vi "Three part faster sub live note on off.vi"() -> ()   [LabVIEW 2009]
uses:
  <vilib>/vision/Image Controls.llb/IMAQ Image.ctl
  <vilib>/userDefined/High Color/IMAQdx.ctl
  <vilib>/Instr/_visa.llb/VISA Configure Serial Port (Instr).vi
  <vilib>/vision/NI_Vision_Development_Module.lvlib
  <vilib>/vision/driver/NI_Vision_Acquisition_Software.lvlib
panel:
  in  "Drum Notes":bool
  out "Image 2":T1(plugin-control)
  in  "VISA resource name":refnum<visa-resource-name>
  out "number":u8 format="%b"
  out "decimal integer string":string
  out "decimal integer string 2":string
  out "decimal integer string 3":string
  out "number 2":u8 format="%b"
  out "number 3":u8 format="%b"
  out "Drum Cluster":T2
  out "Guitar Cluster":T3
  out "Bass Cluster":T4
  in  "Camera":T5="cam0"
  in  "Orange Bass":T6={"Global Rectangle"=[220, 302, 227, 392], "Contours"=[{"ID"=enum."External", "Type"=2, "Coordinates"=[226, 391, 220, 302]}]} {"Contours"."Type" items=["No Selection", "Point", "Line", "Rectangle", "Oval", "Polygon", "Freehand Region", "Annulus", "Unused2", "Unused3", "Broken Line", "Freehand Line", "Rotated Rectangle"]}
  in  "Blue Bass":T6={"Global Rectangle"=[192, 292, 199, 386], "Contours"=[{"ID"=enum."External", "Type"=2, "Coordinates"=[192, 385, 198, 292]}]} {"Contours"."Type" items=["No Selection", "Point", "Line", "Rectangle", "Oval", "Polygon", "Freehand Region", "Annulus", "Unused2", "Unused3", "Broken Line", "Freehand Line", "Rotated Rectangle"]}
  in  "playtime":dbl=90.0
  in  "Orange Guitar":T6={"Global Rectangle"=[587, 282, 628, 378], "Contours"=[{"ID"=enum."External", "Type"=2, "Coordinates"=[627, 377, 587, 282]}]} {"Contours"."Type" items=["No Selection", "Point", "Line", "Rectangle", "Oval", "Polygon", "Freehand Region", "Annulus", "Unused2", "Unused3", "Broken Line", "Freehand Line", "Rotated Rectangle"]}
  in  "Yellow Guitar":T6={"Global Rectangle"=[546, 282, 563, 376], "Contours"=[{"ID"=enum."External", "Type"=2, "Coordinates"=[562, 375, 546, 282]}]} {"Contours"."Type" items=["No Selection", "Point", "Line", "Rectangle", "Oval", "Polygon", "Freehand Region", "Annulus", "Unused2", "Unused3", "Broken Line", "Freehand Line", "Rotated Rectangle"]}
  in  "Green Guitar":T6={"Global Rectangle"=[498, 284, 505, 376], "Contours"=[{"ID"=enum."External", "Type"=2, "Coordinates"=[498, 375, 504, 284]}]} {"Contours"."Type" items=["No Selection", "Point", "Line", "Rectangle", "Oval", "Polygon", "Freehand Region", "Annulus", "Unused2", "Unused3", "Broken Line", "Freehand Line", "Rotated Rectangle"]}
  in  "Blue Guitar":T6={"Global Rectangle"=[569, 290, 594, 372], "Contours"=[{"ID"=enum."External", "Type"=2, "Coordinates"=[593, 371, 569, 290]}]} {"Contours"."Type" items=["No Selection", "Point", "Line", "Rectangle", "Oval", "Polygon", "Freehand Region", "Annulus", "Unused2", "Unused3", "Broken Line", "Freehand Line", "Rotated Rectangle"]}
  in  "Red Guitar":T6={"Global Rectangle"=[526, 284, 530, 370], "Contours"=[{"ID"=enum."External", "Type"=2, "Coordinates"=[529, 369, 526, 284]}]} {"Contours"."Type" items=["No Selection", "Point", "Line", "Rectangle", "Oval", "Polygon", "Freehand Region", "Annulus", "Unused2", "Unused3", "Broken Line", "Freehand Line", "Rotated Rectangle"]}
  in  "Green Bass":T6={"Global Rectangle"=[100, 292, 131, 371], "Contours"=[{"ID"=enum."External", "Type"=2, "Coordinates"=[100, 370, 130, 292]}]} {"Contours"."Type" items=["No Selection", "Point", "Line", "Rectangle", "Oval", "Polygon", "Freehand Region", "Annulus", "Unused2", "Unused3", "Broken Line", "Freehand Line", "Rotated Rectangle"]}
  in  "Red Bass":T6={"Global Rectangle"=[129, 294, 154, 376], "Contours"=[{"ID"=enum."External", "Type"=2, "Coordinates"=[129, 375, 153, 294]}]} {"Contours"."Type" items=["No Selection", "Point", "Line", "Rectangle", "Oval", "Polygon", "Freehand Region", "Annulus", "Unused2", "Unused3", "Broken Line", "Freehand Line", "Rotated Rectangle"]}
  in  "Yellow Bass":T6={"Global Rectangle"=[160, 295, 175, 378], "Contours"=[{"ID"=enum."External", "Type"=2, "Coordinates"=[160, 377, 174, 295]}]} {"Contours"."Type" items=["No Selection", "Point", "Line", "Rectangle", "Oval", "Polygon", "Freehand Region", "Annulus", "Unused2", "Unused3", "Broken Line", "Freehand Line", "Rotated Rectangle"]}
  out "Image Dst Out":T1
  in  "stop":bool
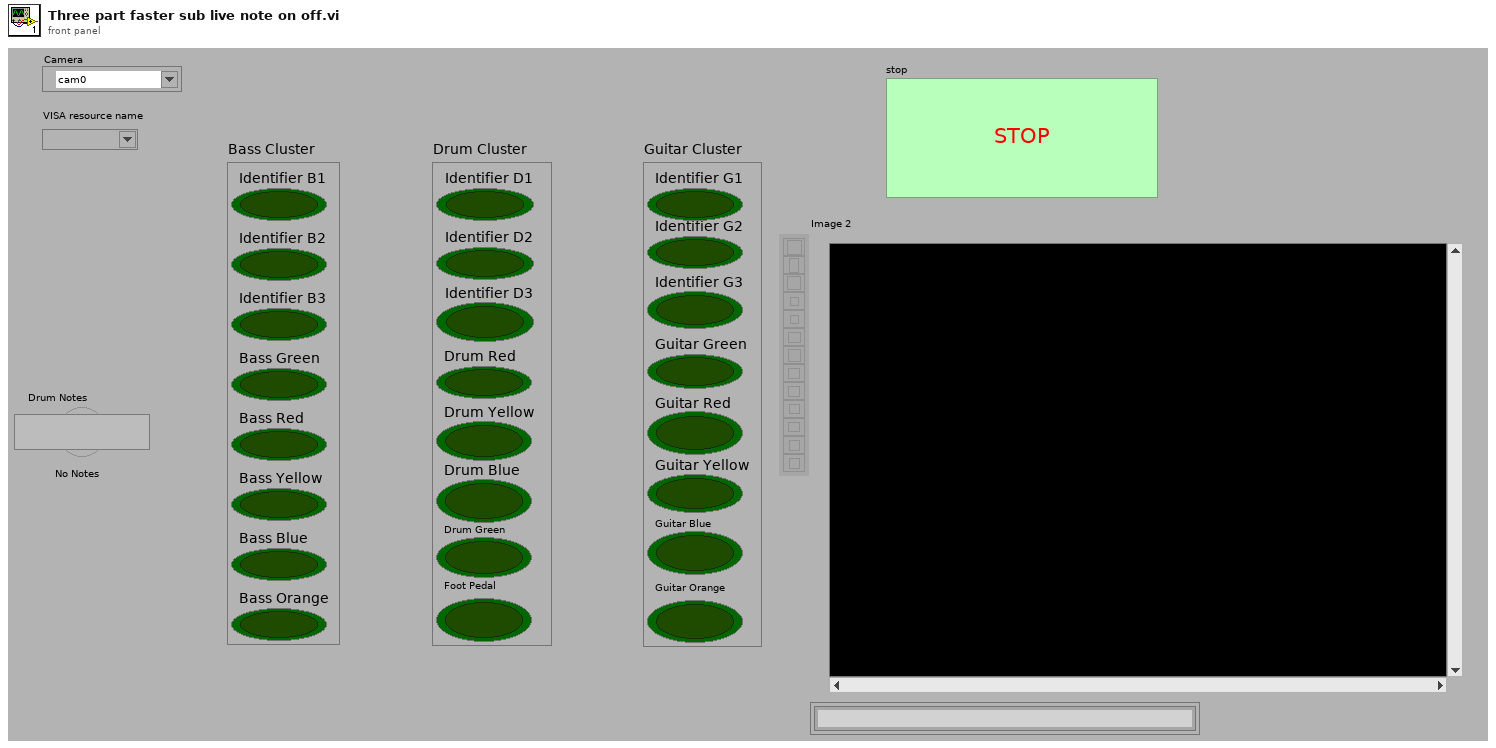
[diagram p1: front panel]
types:
  T1 = typedef "IMAQ Image.ctl" = refnum<image>
  T2 = cluster{"Identifier D1":bool, "Identifier D2":bool, "Identifier D3":bool, "Drum Red":bool, "Drum Yellow":bool, "Drum Blue":bool, "Drum Green":bool, "Foot Pedal":bool}
  T3 = cluster{"Identifier G1":bool, "Identifier G2":bool, "Identifier G3":bool, "Guitar Green":bool, "Guitar Red":bool, "Guitar Yellow":bool, "Guitar Blue":bool, "Guitar Orange":bool}
  T4 = cluster{"Identifier B1":bool, "Identifier B2":bool, "Identifier B3":bool, "Bass Green":bool, "Bass Red":bool, "Bass Yellow":bool, "Bass Blue ":bool, "Bass Orange":bool}
  T5 = typedef "IMAQdx.ctl" = refnum<k21>
  T6 = cluster{"Global Rectangle":i32[], "Contours":cluster{"ID":enum32{"External", "Internal"}, "Type":u32, "Coordinates":i32[]}[]}
  T7 = typedef "Image Type" = u32
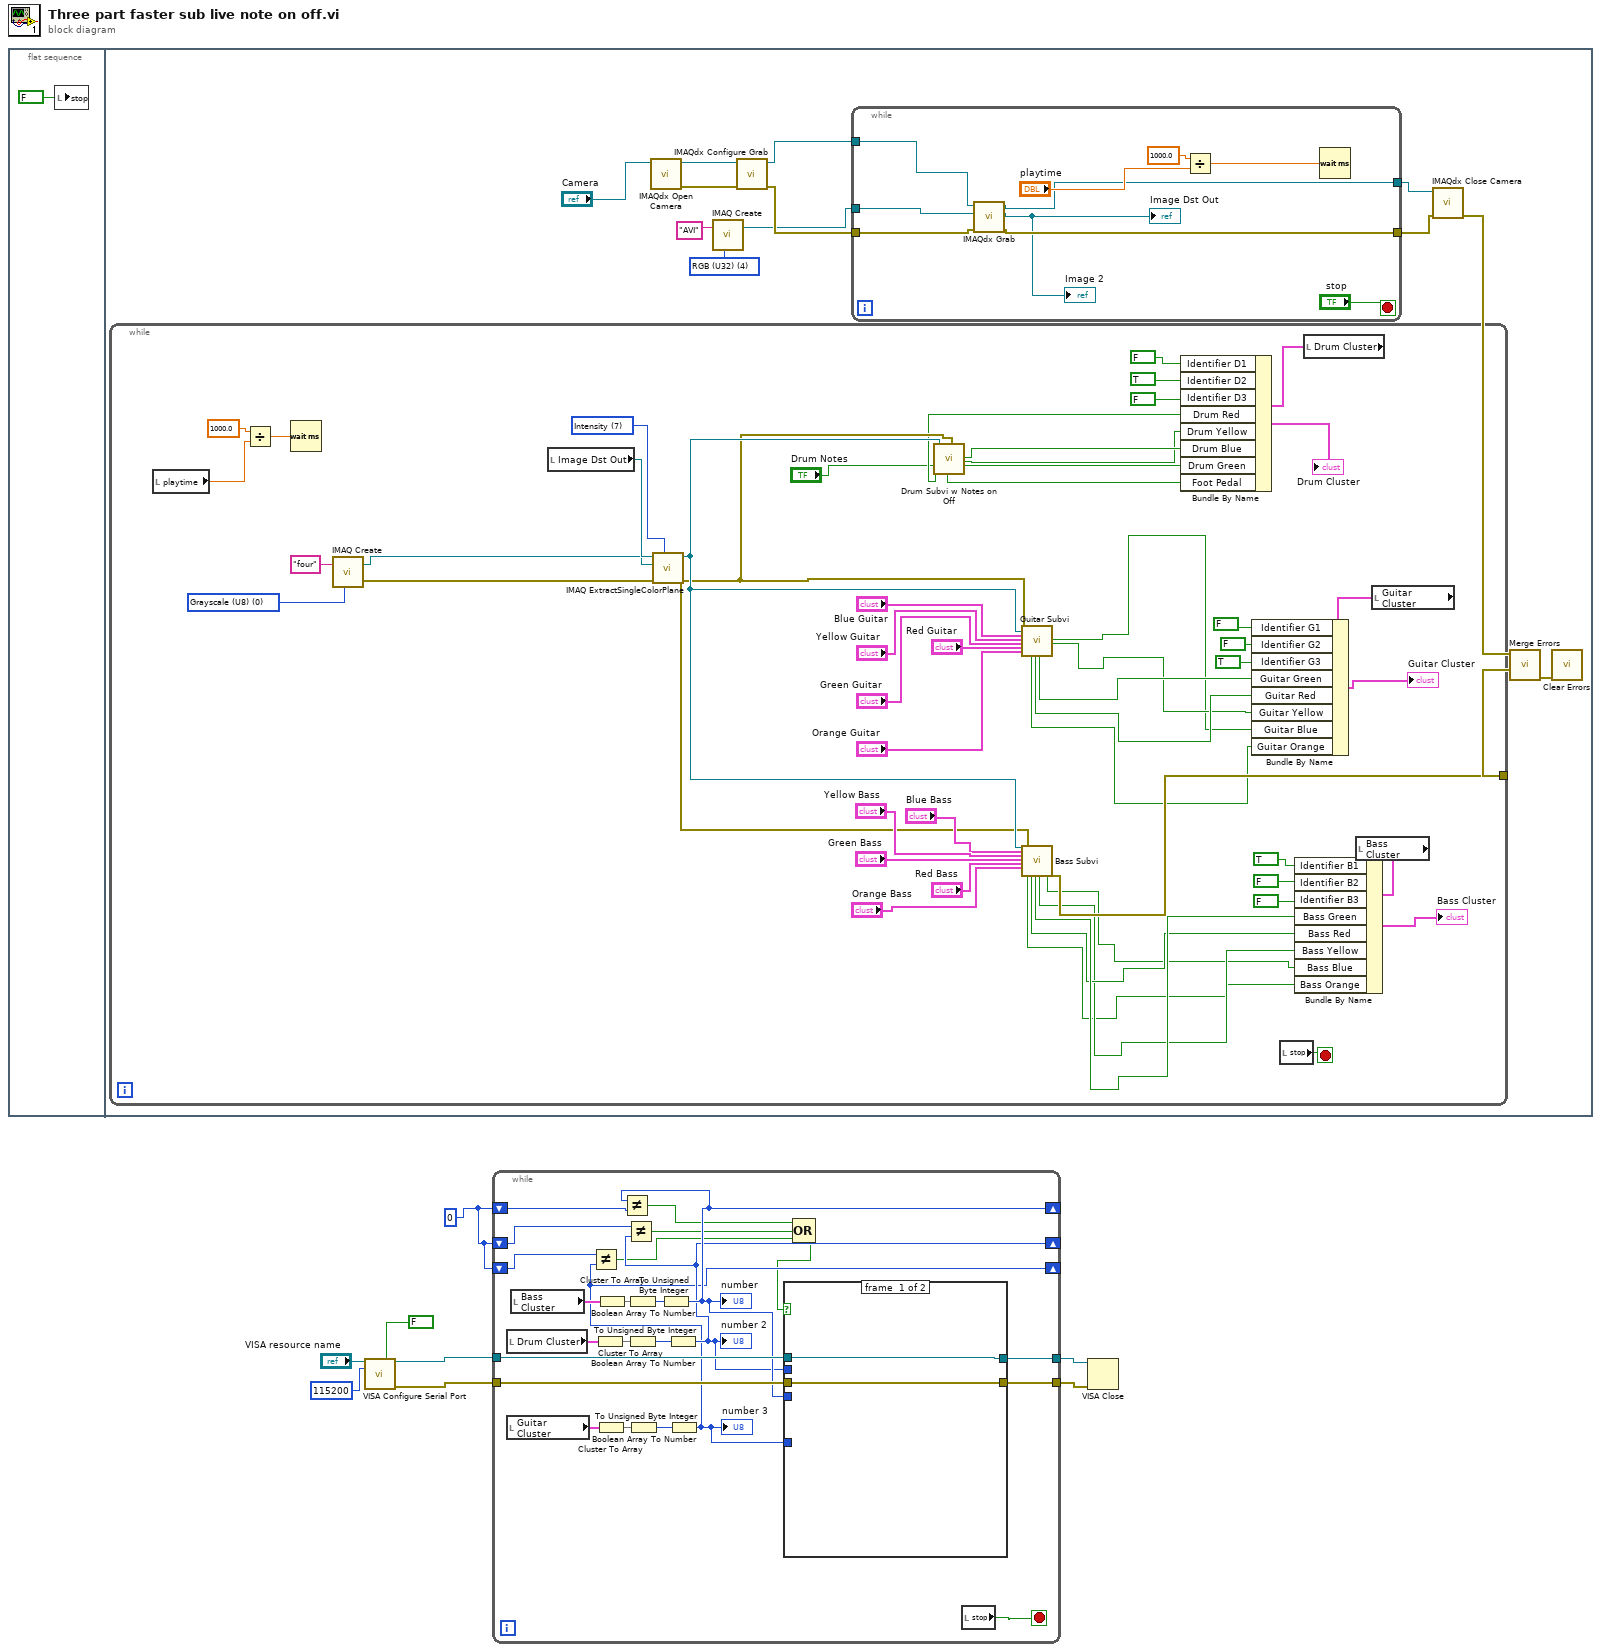
[diagram p0: block diagram]
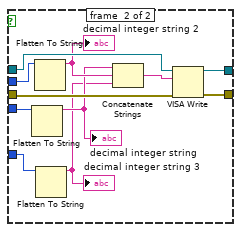
[diagram p2: hidden frame]
diagram:
  w1 = u8 0
  n1 = flat-sequence {
    frame #0 {
      n2 = local write "stop"(FALSE ("stop")) -> ()
    }
    frame #1 {
      w20 = T7 4 items=["Grayscale (U8)", "Grayscale (I16)", "Grayscale (SGL)", "Complex (CSG)", "RGB (U32)", "HSL (U32)", "RGB (U64)", "Grayscale (U16)"] ("Image Type")
      n3 = while {
        tunnel: [w66] -> w21
        stop <- w75 stop-if-true
        w71 = T7 0 items=["Grayscale (U8)", "Grayscale (I16)", "Grayscale (SGL)", "Complex (CSG)", "RGB (U32)", "HSL (U32)", "RGB (U64)", "Grayscale (U16)"] ("Image Type")
        w76 = 7 items=["Red", "Green", "Blue", "Hue", "Saturation", "Luminance", "Value", "Intensity"] ("Color Plane")
        n4 = local read "playtime"() -> (w60:dbl)
        n5 = Divide(x=1000.0, y=w60) -> (x/y=w74:dbl)
        n6 = Wait (ms)(milliseconds to wait=w74) -> ()  [unwired: 1 out]
        n7 = call "IMAQ Create"("Image Name"="four", "Image Type"=w71) -> ("New Image"=w24:T1, "error out"=w23:errorcluster)  [unwired: 3 in]
        n8 = local read "Image Dst Out"() -> (w72:T1)
        n9 = call "IMAQ ExtractSingleColorPlane"("Color Plane"=w76, "error in (no error)"=w23, "Image Dst"=w24, "Image Src"=w72) -> ("error out"=w31:errorcluster, "Image Dst Out"=w32:T1)  [unwired: 6 out]
        n10 = call "Drum Subvi w Notes on Off.vi"("Drum Notes On/Off"="Drum Notes", "Image Dst Out"=w32, "error out"=w31) -> ("Red Drum"=w26:bool, "Foot Pedal"=w27:bool, "Blue Drum 2"=w30:bool, "Yellow Drum"=w28:bool, "Green Drum"=w29:bool)  [unwired: 16 in, 4 out]
        n11 = call "Guitar Subvi.vi"("error out"=w31, "Image Dst Out"=w32, "Blue Guitar 2"="Blue Guitar", "Yellow Guitar 2"="Yellow Guitar", "Green Guitar 2"="Green Guitar", "Red Guitar 2"="Red Guitar", "Orange Guitar 2"="Orange Guitar") -> ("Orange Guitar LED"=w38:bool, "Red Guitar LED"=w41:bool, "Green Guitar LED"=w42:bool, "Blue Guitar LED"=w39:bool, "Yellow Guitar LED"=w40:bool)  [unwired: 16 in]
        n12 = call "Bass Subvi.vi"("Image Dst Out"=w32, "Blue Bass 2"="Blue Bass", "Yellow Bass 2"="Yellow Bass", "Green Bass 2"="Green Bass", "Red Bass 2"="Red Bass", "Orange Bass 2"="Orange Bass", "error out"=w31) -> ("Orange Bass LED"=w48:bool, "Red Bass LED"=w51:bool, "Green Bass LED"=w52:bool, "Yellow Bass LED"=w50:bool, "Blue Bass LED"=w49:bool, "error out 2"=w66:errorcluster)  [unwired: 15 in]
        n13 = local read "stop"() -> (w75:bool)
        n14 = local read "Drum Cluster"() -> (w36:T2)
        n15 = Bundle By Name(cluster=w36, "Identifier D1"=FALSE, "Identifier D2"=TRUE ("element"), "Identifier D3"=FALSE ("element"), "Drum Red"=w26, "Drum Yellow"=w28, "Drum Blue"=w30, "Drum Green"=w29, "Foot Pedal"=w27) -> (→"Drum Cluster":T2)
        n16 = local read "Bass Cluster"() -> (w57:T4)
        n17 = Bundle By Name(cluster=w57, "Identifier B1"=TRUE, "Identifier B2"=FALSE ("element"), "Identifier B3"=FALSE ("element"), "Bass Green"=w52, "Bass Red"=w51, "Bass Yellow"=w50, "Bass Blue"=w49, "Bass Orange"=w48) -> (→"Bass Cluster":T4)
        n18 = local read "Guitar Cluster"() -> (w46:T3)
        n19 = Bundle By Name(cluster=w46, "Identifier G1"=FALSE ("element"), "Identifier G2"=FALSE ("element"), "Identifier G3"=TRUE ("element"), "Guitar Green"=w42, "Guitar Red"=w41, "Guitar Yellow"=w40, "Guitar Blue"=w39, "Guitar Orange"=w38) -> (→"Guitar Cluster":T3)
      }
      n20 = call <vilib>:"IMAQdx Open Camera.vi"("Session In"="Camera") -> ("error out"=w18:errorcluster, "Session Out"=w17:T5)  [unwired: 9 in]
      n21 = call "IMAQ Create"("Image Name"="AVI", "Image Type"=w20) -> ("New Image"=w13:T1)  [unwired: 3 in, 1 out]
      n22 = call <vilib>:"IMAQdx Configure Grab.vi"("error in"=w18, "Session In"=w17) -> ("error out"=w14:errorcluster, "Session Out"=w15:T5)  [unwired: 8 in]
      n23 = while {
        tunnel: w13 -> [w80]
        tunnel: w14 -> [w82]
        tunnel: [w79] -> w10
        tunnel: [w78] -> w12
        tunnel: w15 -> [w81]
        stop <- "stop" stop-if-true
        n24 = call <vilib>:"IMAQdx Grab.vi"("error in"=w82, "Image In"=w80, "Session In"=w81) -> ("error out"=w78:errorcluster, "Image Out"=→"Image Dst Out" →"Image 2":T1, "Session Out"=w79:T5)  [unwired: 5 in, 1 out]
        n25 = Divide(x=1000.0, y="playtime") -> (x/y=w85:dbl)
        n26 = Wait (ms)(milliseconds to wait=w85) -> ()  [unwired: 1 out]
      }
      n27 = call <vilib>:"IMAQdx Close Camera.vi"("error in"=w12, "Session In"=w10) -> ("error out"=w11:errorcluster)  [unwired: 9 in]
      n28 = call <vilib>:"Merge Errors.vi"("error in 3 (no error)"=w21, "error in 1 (no error)"=w11) -> ("error out"=w22:errorcluster)  [unwired: 5 in]
      n29 = call <vilib>:"Clear Errors.vi"("error in (no error)"=w22) -> ()  [unwired: 6 in, 1 out]
    }
  }
  n30 = call-poly "VISA Configure Serial Port"("VISA resource name"="VISA resource name", "Enable Termination\nChar (T)"=FALSE ("Enable Termination\nChar (T)"), "baud rate (9600)"=u32 115200) -> ("VISA resource name out"=w8:refnum<visa-resource-name>, "error out"=w3:errorcluster)  [unwired: 11 in]
  n31 = while {
    tunnel: w8 -> [w110]
    tunnel: [w109] -> w7
    tunnel: w3 -> [w108]
    tunnel: [w107] -> w2
    shift-right: [w99] -> _
    shift-left: w1 -> [w98]
    shift-right: [w97] -> _
    shift-left: w1 -> [w96]
    shift-right: [w91] -> _
    shift-left: w1 -> [w92]
    stop <- w102 stop-if-true
    n32 = local read "Drum Cluster"() -> (w104:T2)
    n33 = local read "Guitar Cluster"() -> (w94:T3)
    n34 = local read "Bass Cluster"() -> (w103:T4)
    n35 = Cluster To Array(cluster=w104) -> (array=w105:bool[])
    n36 = Cluster To Array(cluster=w94) -> (array=w93:bool[])
    n37 = Cluster To Array(cluster=w103) -> (array=w106:bool[])
    n38 = Boolean Array To Number(Boolean array=w106) -> (number=w101:u32)
    n39 = Boolean Array To Number(Boolean array=w105) -> (number=w100:u32)
    n40 = Boolean Array To Number(Boolean array=w93) -> (number=w95:u32)
    n41 = To Unsigned Byte Integer(number=w101) -> (unsigned 8bit integer=w99:u8)
    "number" <- w99
    n42 = Not Equal?(x=w99, y=w98) -> (x != y?=w89:bool)
    n43 = To Unsigned Byte Integer(number=w100) -> (unsigned 8bit integer=w97:u8)
    "number 2" <- w97
    n44 = Not Equal?(x=w96, y=w97) -> (x != y?=w88:bool)
    n45 = To Unsigned Byte Integer(number=w95) -> (unsigned 8bit integer=w91:u8)
    "number 3" <- w91
    n46 = Not Equal?(x=w92, y=w91) -> (x != y?=w87:bool)
    n47 = Compound Arithmetic op=OR(w89, w88, w87) -> (w90:bool)
    n48 = case shown="True" w90 {
      tunnel: w110 -> [w112 w123]
      tunnel: [w112 w122] -> w109
      tunnel: w99 -> [_ w116]
      tunnel: w108 -> [w111 w121]
      tunnel: [w111 w120] -> w107
      tunnel: w97 -> [_ w118]
      tunnel: w91 -> [_ w113]
      frame #0 {
      }
      frame #1 {
        n49 = Flatten To String(anything=w116) -> (data string=w115:string)  [unwired: 3 in, 2 out]
        "decimal integer string" <- w115
        n50 = Flatten To String(anything=w118) -> (data string=w117:string)  [unwired: 3 in, 2 out]
        "decimal integer string 2" <- w117
        n51 = Flatten To String(anything=w113) -> (data string=w114:string)  [unwired: 3 in, 2 out]
        "decimal integer string 3" <- w114
        n52 = Concatenate Strings(w115, w117, w114) -> (w119:string)
        n53 = VISA Write(VISA resource name=w123, write buffer=w119, error in (no error)=w121) -> (VISA resource name out=w122:refnum<visa-resource-name>, error out=w120:errorcluster)  [unwired: 1 out]
      }
    }
    n54 = local read "stop"() -> (w102:bool)
  }
  n55 = VISA Close(VISA resource name=w7, error in (no error)=w2) -> ()  [unwired: 1 out]
